vi "test simple.vi"() -> ()   [LabVIEW 2013, in "infolib.lvlib"]
uses:
  infolib.lvlib
  Add matrix polymorph parts/2D EXT.vi
  Get key polymorph parts/GetI64.vi
  Get matrix polymorph parts/Get 2D EXT.vi
panel:
  in  "matrix":dbl[][](array[numeric])
  in  "matrix key":string="somematrix"
  out "reading from\ninfo file ok?":bool
  in  "value 2":i64=2
  in  "value after long insert":i64=5
  in  "key after long insert":string="key after long insert"
  in  "key 1":string="number test1 (A)"
  in  "key 2":string="number test2 $\\"
  in  "to insert":string="TEST string\nthat will be \ninserted"
  in  "sections 2":string[](array[string])=["adc u calibration data"]
  out "joining two info strings:":string
  in  "sections":string[](array[string])=["section 1", "section 2"]
  in  "value 1":i64=1
  out "section do not exist, section is set":string
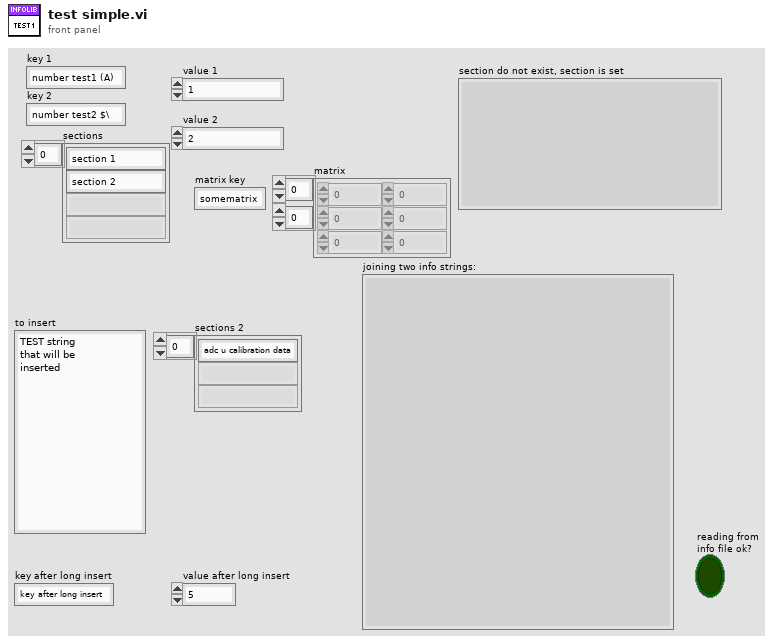
[diagram p1: front panel]
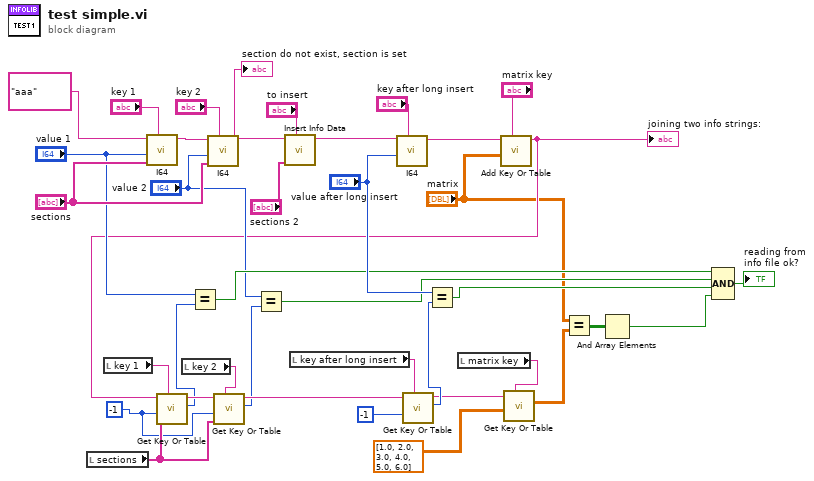
[diagram p0: block diagram]
diagram:
  w24 = i64 -1 ("values")
  n1 = local read "sections"() -> (w25:string[])
  n2 = local read "key 1"() -> (w28:string)
  n3 = call "I64.vi"("key description"="key 1", "sections"="sections", "numeric"="value 1", "info data"="aaa") -> ("info data out"=w35:string)  [unwired: 6 in, 1 out]
  n4 = local read "key 2"() -> (w26:string)
  n5 = call "I64.vi"("key description"="key 2", "sections"="sections", "numeric"="value 2", "info data"=w35) -> ("info data out"=w33:string)  [unwired: 6 in, 1 out]
  "section do not exist, section is set" <- w33
  n6 = call "Insert Info Data.vi"("info data to insert"="to insert", "sections"="sections 2", "info data"=w33) -> ("info data out"=w32:string)  [unwired: 7 in, 1 out]
  n7 = local read "key after long insert"() -> (w11:string)
  n8 = call "I64.vi"("key description"="key after long insert", "numeric"="value after long insert", "info data"=w32) -> ("info data out"=w10:string)  [unwired: 7 in, 1 out]
  n9 = local read "matrix key"() -> (w5:string)
  n10 = call-poly "Add Key Or Table.vi"("key description"="matrix key", "numeric"="matrix", "info data"=w10) -> ("info data out"=w8:string)  [unwired: 7 in, 1 out]
  "joining two info strings:" <- w8
  n11 = call-poly "Get Key Or Table.vi"("key description"=w28, "sections"=w25, "numeric"=w24, "info data"=w8) -> ("value"=w19:i64, "info data out"=w27:string)  [unwired: 5 in, 1 out]
  n12 = Equal?(x="value 1", y=w19) -> (x = y?=w16:bool)
  n13 = call-poly "Get Key Or Table.vi"("key description"=w26, "sections"=w25, "numeric"=w24, "info data"=w27) -> ("value"=w18:i64, "info data out"=w23:string)  [unwired: 5 in, 1 out]
  n14 = Equal?(x="value 2", y=w18) -> (x = y?=w15:bool)
  n15 = call-poly "Get Key Or Table.vi"("key description"=w11, "numeric"=i64 -1 ("values"), "info data"=w23) -> ("value"=w21:i64, "info data out"=w6:string)  [unwired: 6 in, 1 out]
  n16 = Equal?(x="value after long insert", y=w21) -> (x = y?=w14:bool)
  n17 = call-poly "Get Key Or Table.vi"("key description"=w5, "numeric"=dbl[][] [[1.0, 2.0], [3.0, 4.0], [5.0, 6.0]] ("matrix 2"), "info data"=w6) -> ("value"=w4:ext[][])  [unwired: 6 in, 2 out]
  n18 = Equal?(x="matrix", y=w4) -> (x = y?=w2:bool[][])
  n19 = And Array Elements(Boolean array=w2) -> (logical AND=w1:bool)
  n20 = Compound Arithmetic op=AND(w16, w15, w14, w1) -> (→"reading from\ninfo file ok?":bool)
